vi "Utility Format Pressure Limit.vi"(8 "error in (no error)":errorcluster, 10 "Pressure Limit":i32, 11 "Pressure Limit Command":string="UP") -> (0 "error out":errorcluster, 3 "Formatted Command":string)   [LabVIEW 2020, in "ChromTech Series III Pump.lvlib"]
doc: "Formats the pressure limit given into the message format \"XXxxxx\", where \"XX\" is the command and \"xxxx\" is the four-digit pressure limit given. No error checking is performed to ensure pressure limits are in a valid range, so be sure to consult the manual and set proper pressure limits for your pump head."
uses:
  <instrlib>/RxnRover/ChromtechSeriesIIIDriver/ChromTech Series III Pump.lvlib
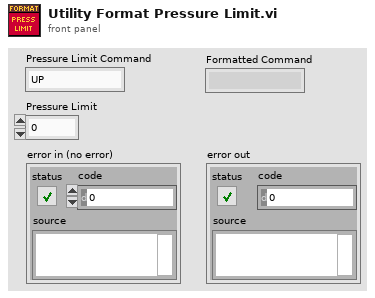
[diagram p1: front panel]
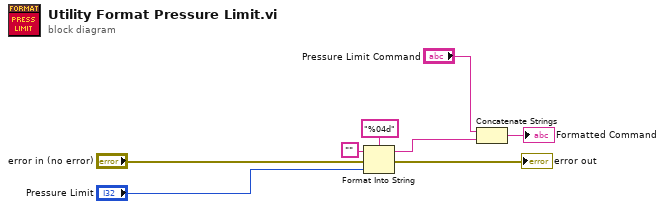
[diagram p0: block diagram]
diagram:
  n1 = Format Into String(format string="%04d", initial string="", error in="error in (no error)", "Pressure Limit") -> (resulting string=w3:string, error out=→"error out":errorcluster)
  n2 = Concatenate Strings("Pressure Limit Command", w3) -> (→"Formatted Command":string)
